vi "Mindsensors AngleSensor Config.vi"(10 "Node Data":T1, 11 "NXT":T2) -> ()   [LabVIEW 2010]
uses:
  <vilib>/NXT/Subs/LVHSConnector.ctl
  Datatypes/Node.ctl
  UI Controls/PlugInControls/Pluginbackground.ctl
  <vilib>/Utility/miscctls.llb/LVPointTypeDef.ctl
  <vilib>/NXT/Block Support/HWPage.SensorMode.ctl
  <vilib>/NXT/Block Support/HWPage.SensorType.ctl
  ConvertNodeAddrSensor.vi
panel:
  out "Raw Value (half degree)":i32
  out "RPM":i16
  in  "Device Addr":i32 format="%.0x"
  out "Angle (degrees)":i32
  out "?":u8
  out "number":i8
  in  "Device Address":string
  in  "NXT Port":string
  in  "Name":string
  out "Headline":string="Type (auto populated)"
  in  "Sensor Parameters":string
  in  "Instance Specific Data":cluster{"Example Data":dbl}
  in  "Reset":bool
  in  "Save":bool
  in  "Stop":bool
  out "Background":T3=TRUE
  # "Sensor Values"
  # "<- No controls below this line"
  # "Common controls such as Buttons, Rings, Sliders, Graphs, Decorations, etc can be found in the <labview>\\Targets\\NI\\NXT\\NXT Toolkit\\Schematic Editor\\UI Controls\\Plugin Controls\\ folder. Use these controls when possible to ensure a consistent look and feel with LabVIEW Education Edition."
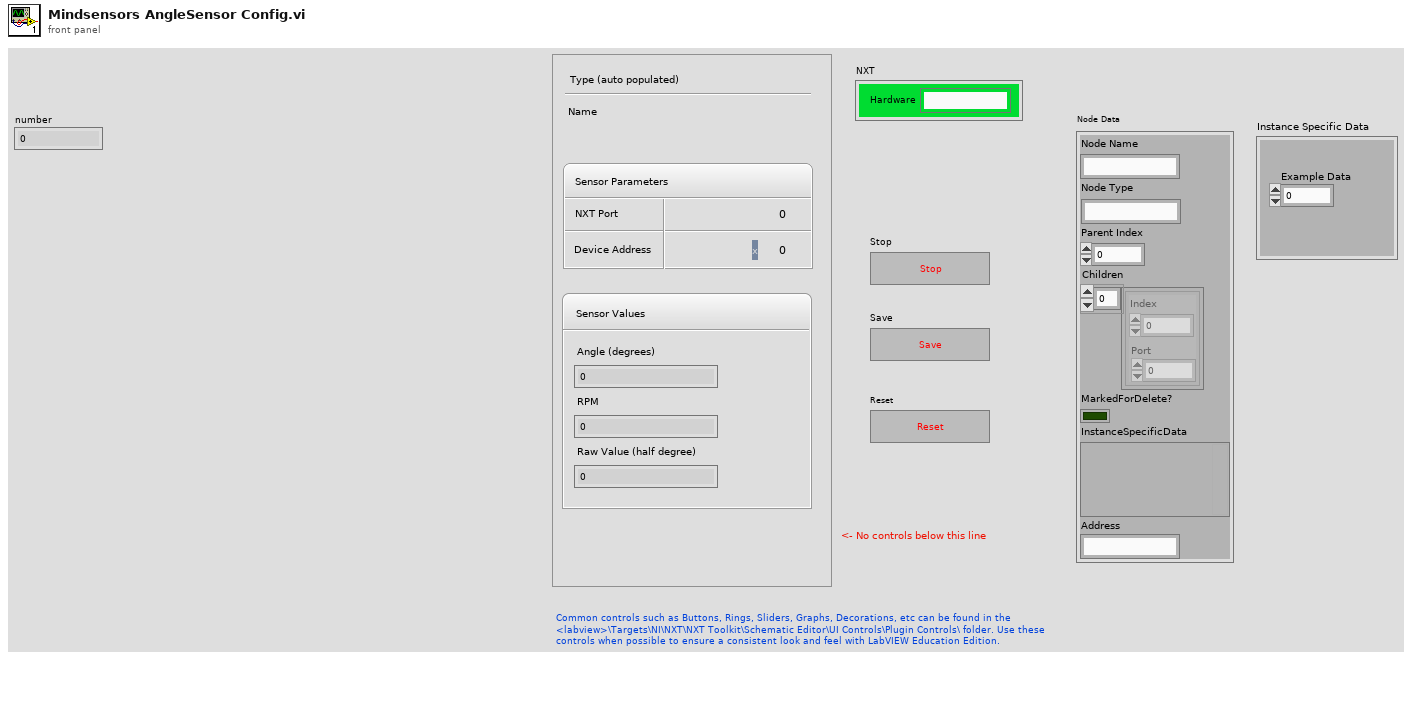
[diagram p1: front panel]
types:
  T1 = typedef "Node.ctl" = cluster{"Node Name":string, "Node Type":string, "Parent Index":i16, "Children":cluster{"Index":u16, "Port":u16}[], "MarkedForDelete?":bool, "InstanceSpecificData":variant, "Address":string}
  T2 = typedef "LVHSConnector.ctl" = cluster{"Hardware":string, "Flattened String":string}
  T3 = typedef "Pluginbackground.ctl" = bool
  T4 = typedef "LVPointTypeDef.ctl" = cluster{"Horizontal":i16, "Vertical":i16}
  T5 = enum8{"Enabled", "Disabled", "Disabled and Grayed Out"}
  T6 = typedef "HWPage.SensorMode.ctl" = u8
  T7 = typedef "HWPage.SensorType.ctl" = u8
  T8 = typedef "NXT_InputPort.ctl" = u8
  T9 = typedef "nxt.ctl" = cluster{"nxtHandle":u32, "fileHandle":u32, "fileIterHandle":u32, "moduleHandle":u32, "modIterHandle":u32, "nxtIterHandle":u32}
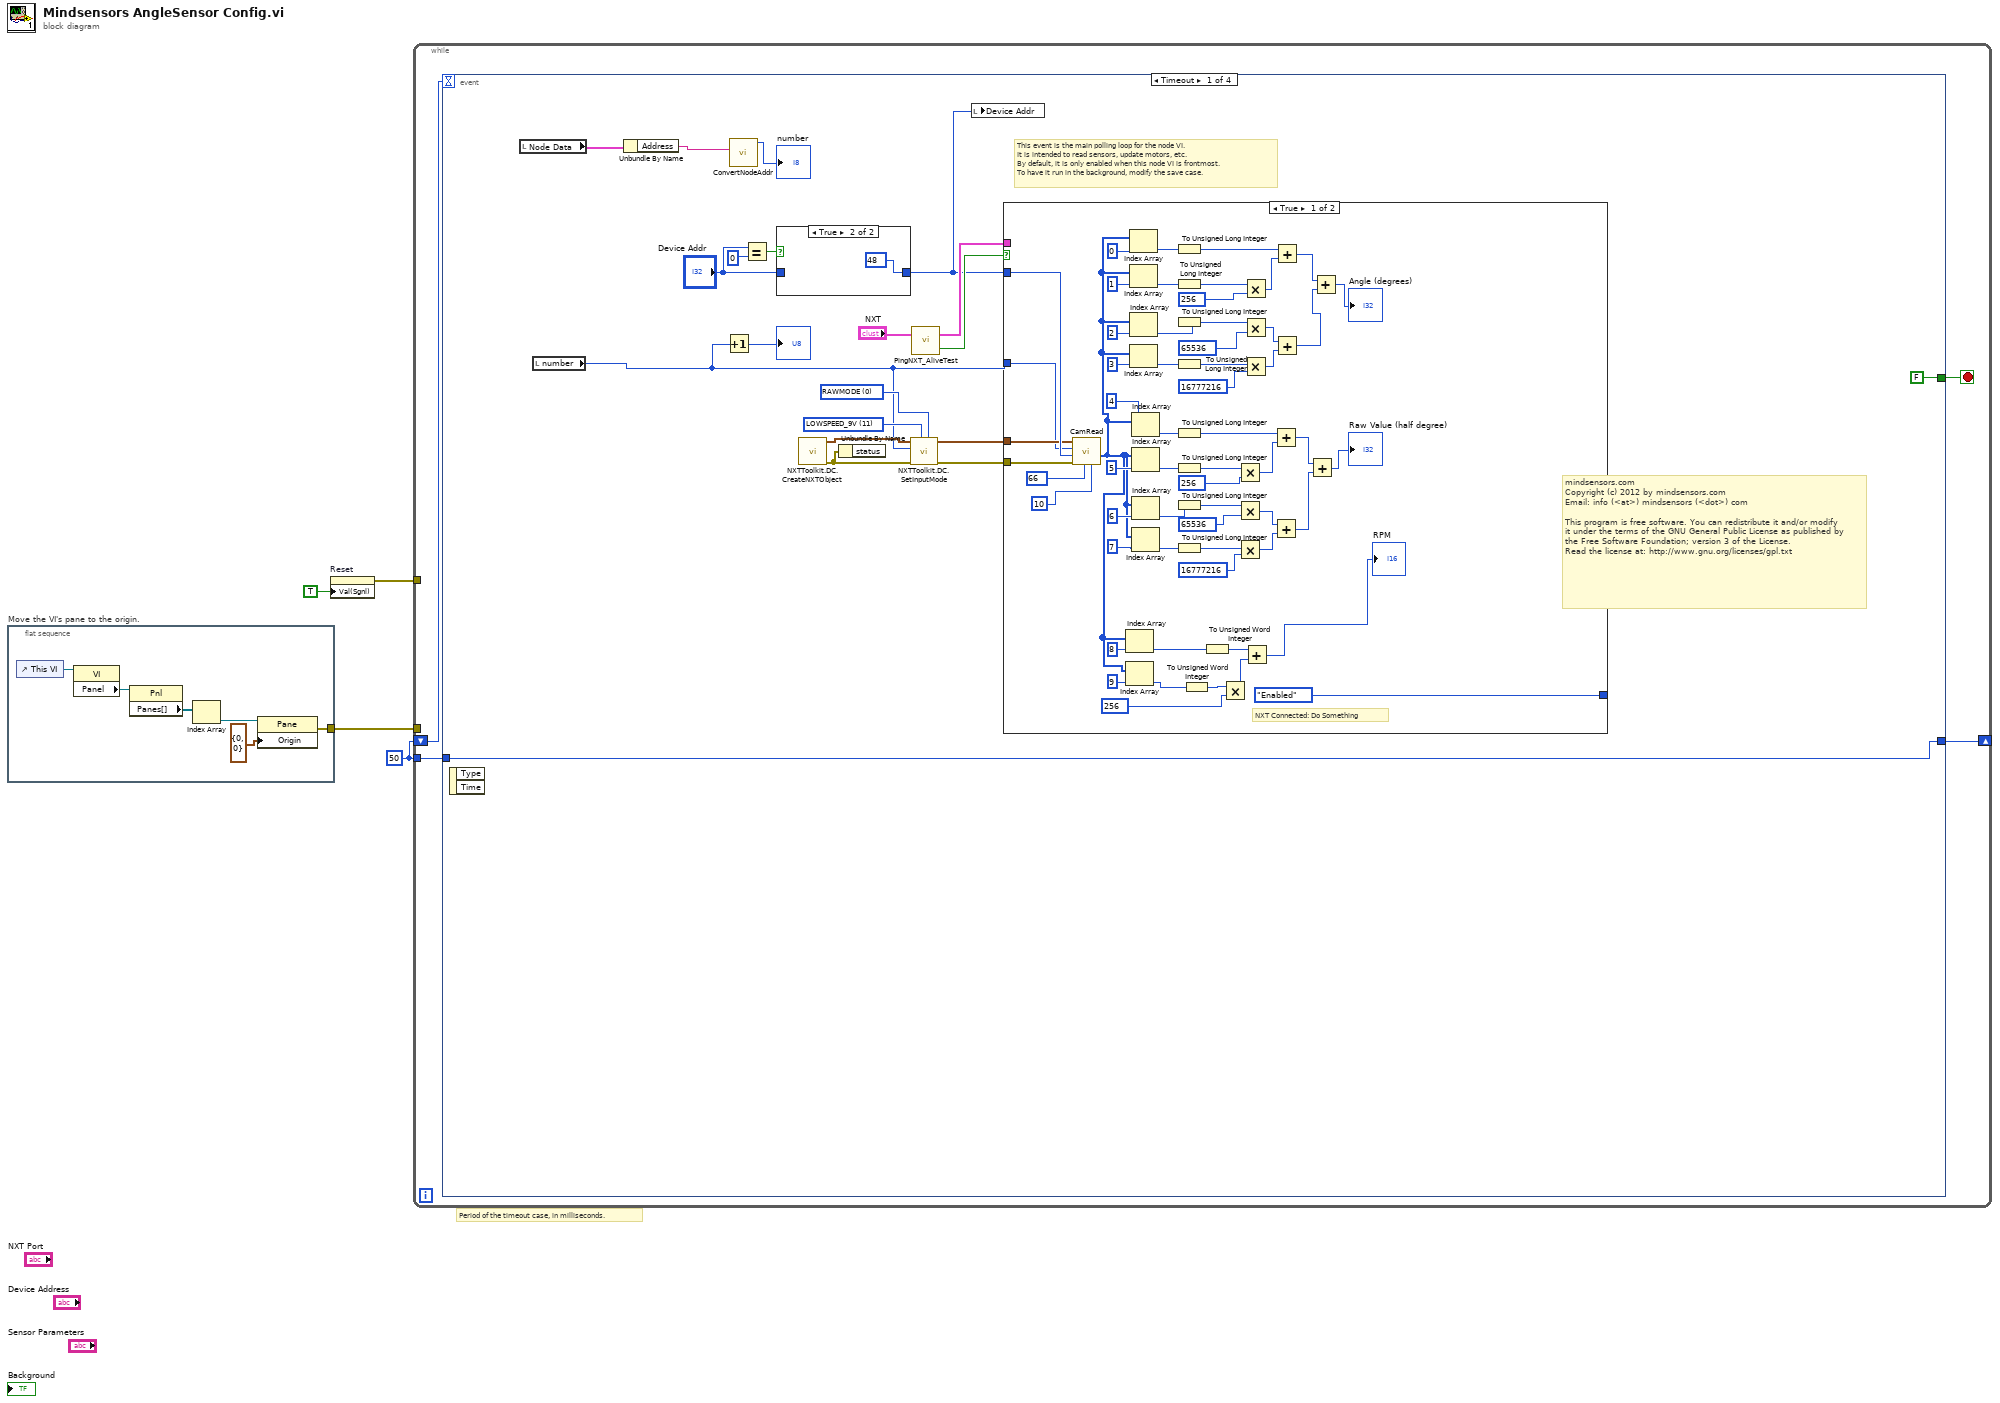
[diagram p0: block diagram]
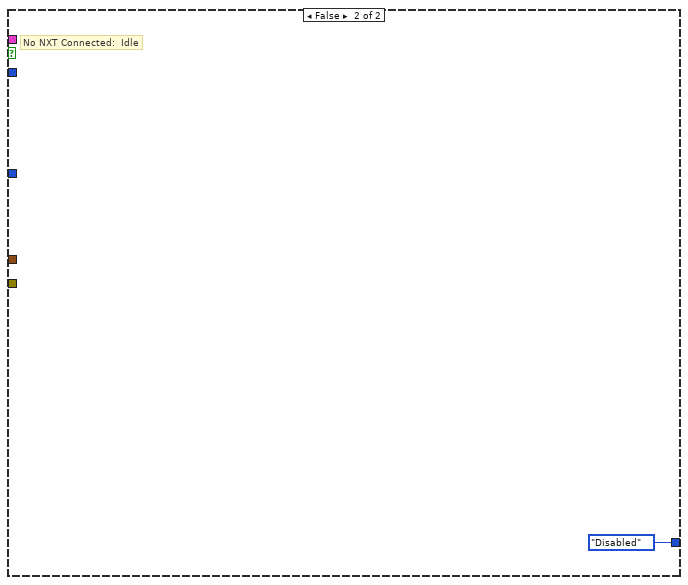
[diagram p3: hidden frame]
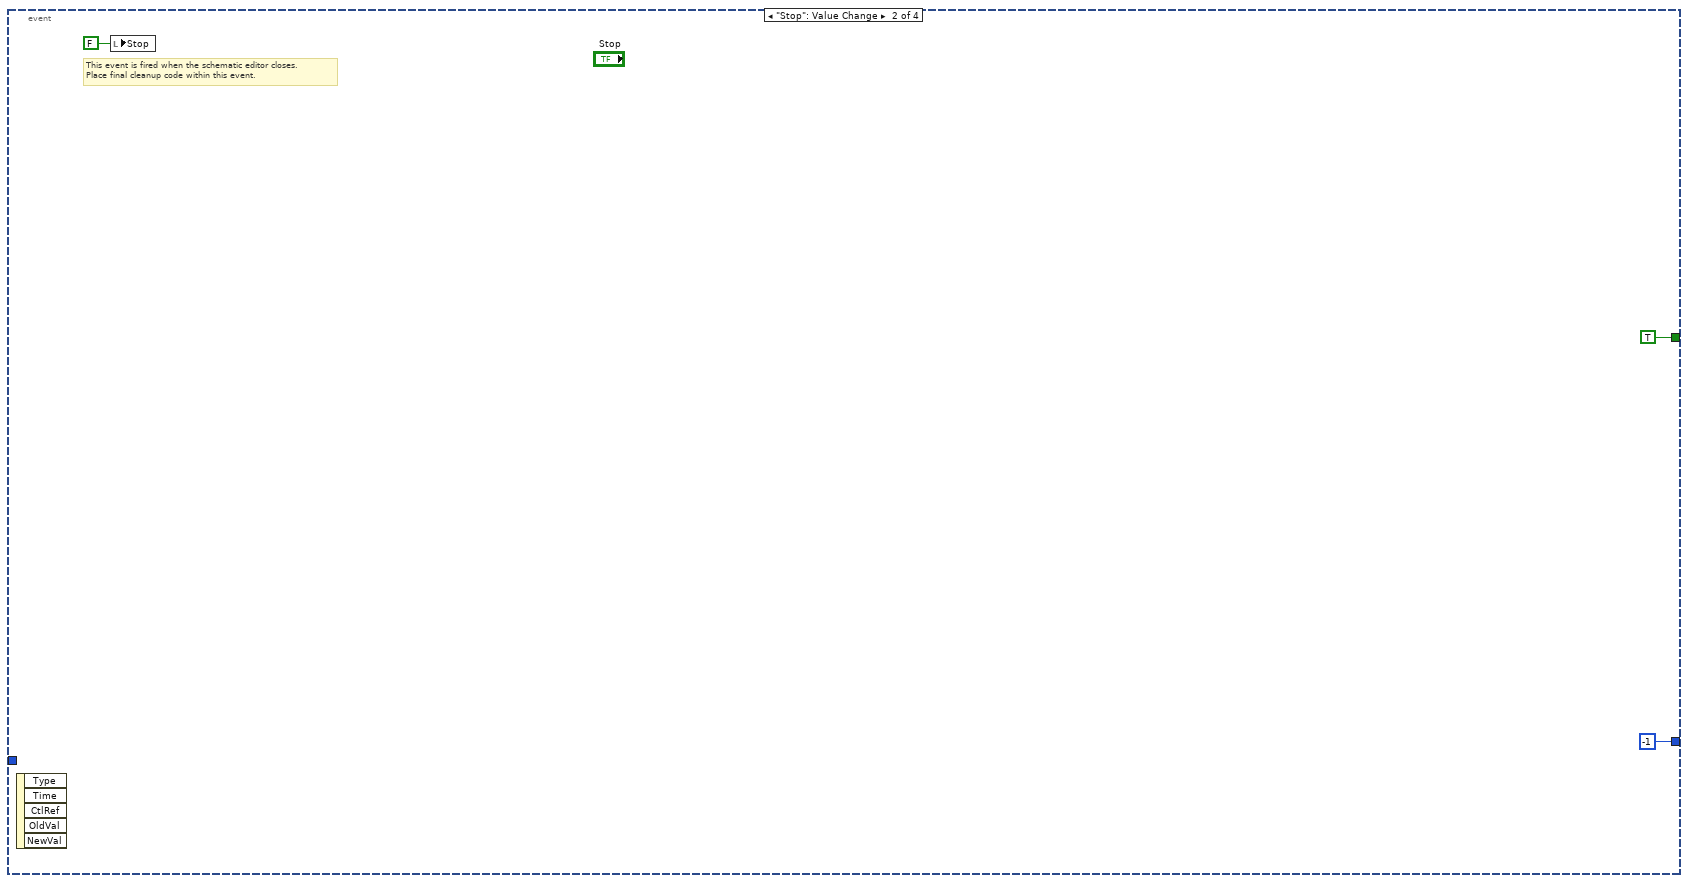
[diagram p4: hidden frame]
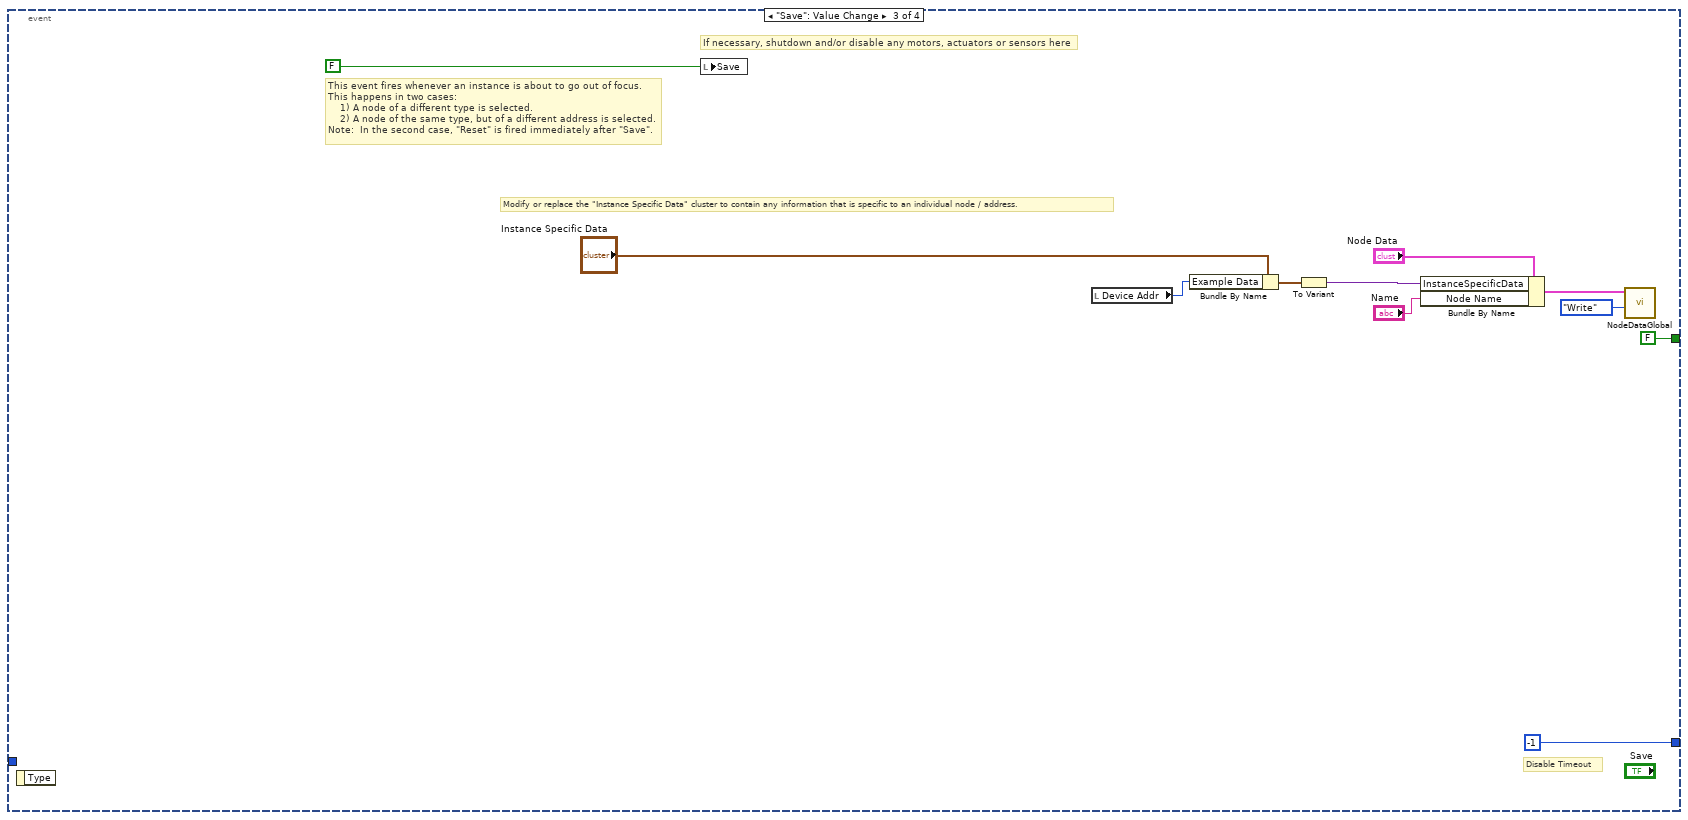
[diagram p5: hidden frame]
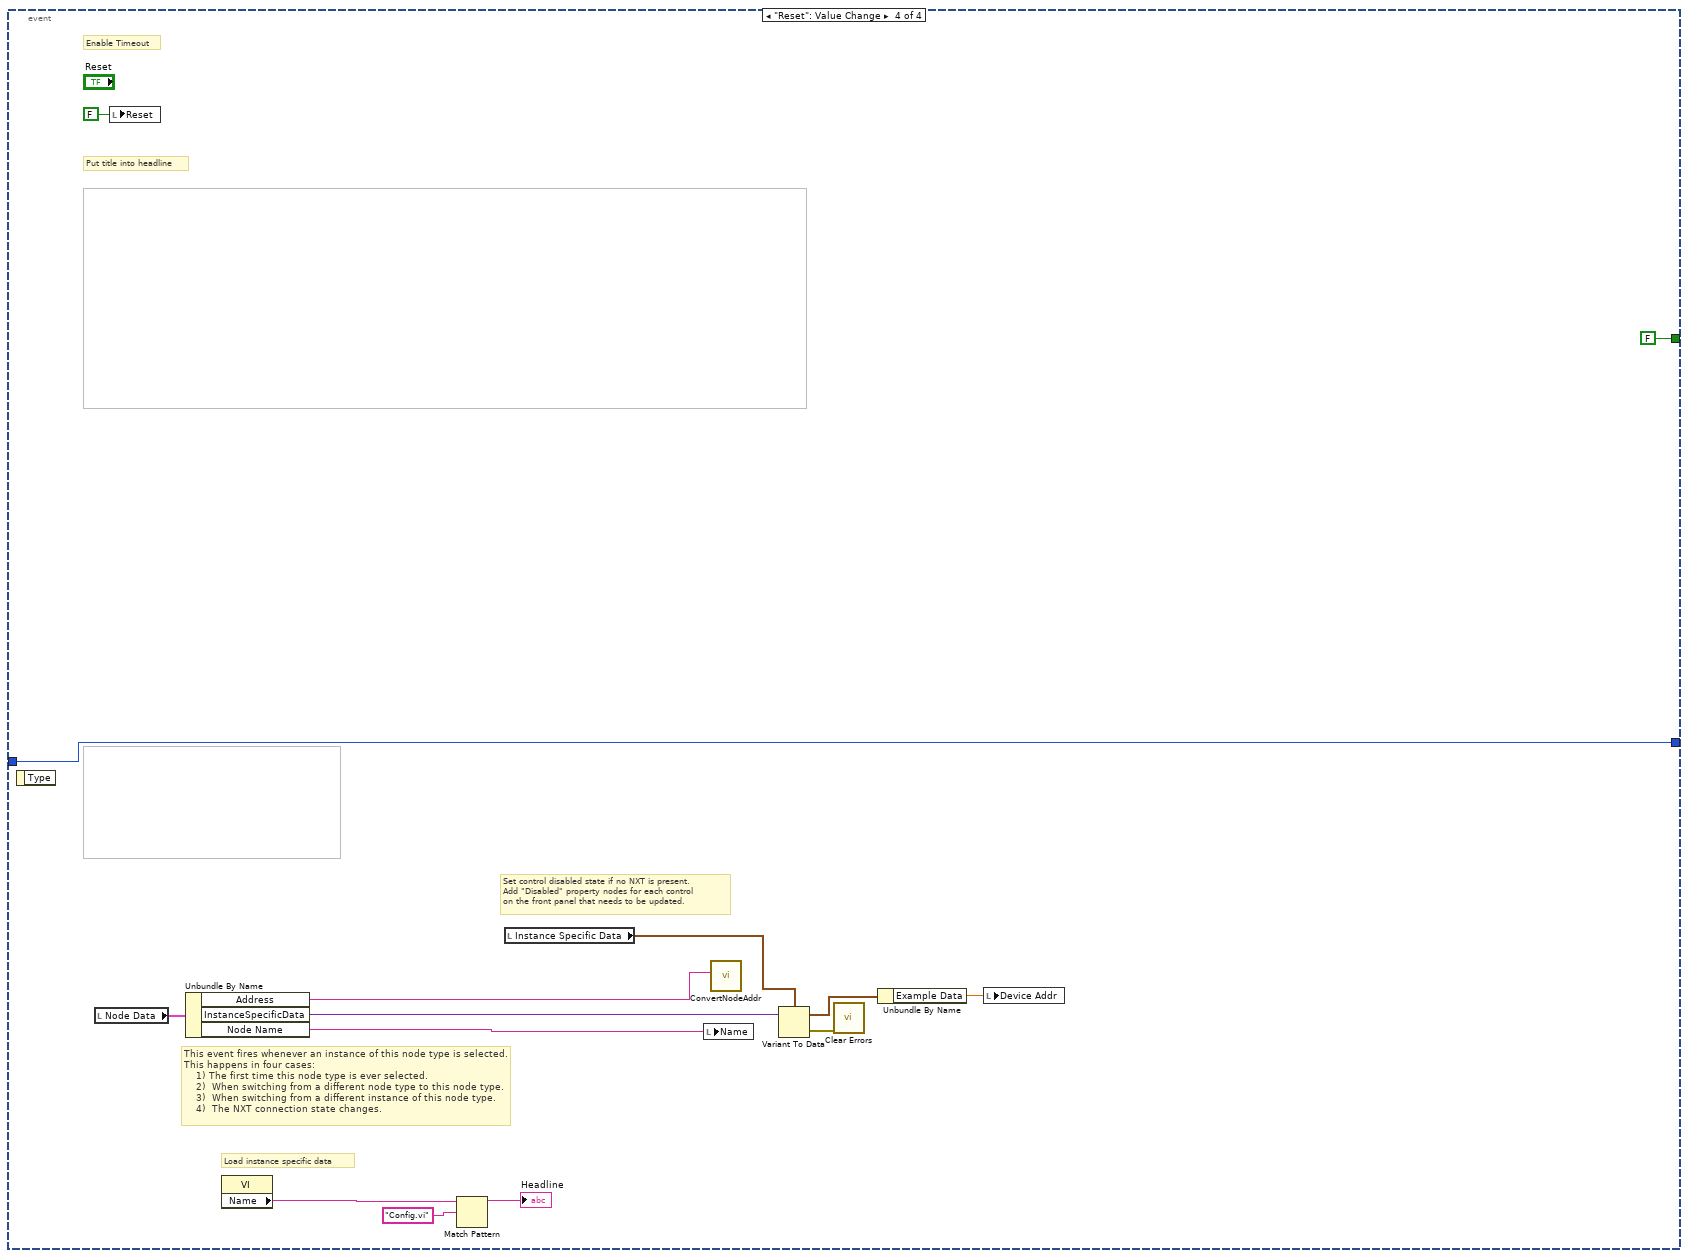
[diagram p6: hidden frame]
diagram:
  w2 = 50
  # "Period of the timeout case, in milliseconds."
  n1 = flat-sequence "Move the VI's pane to the origin." {
    tunnel: [w5] -> w1
    frame #0 {
      n2 = control-ref of="This VI"() -> (w6:refnum<vi>)
      n3 = property class="VI"(reference=w6) -> ("Panel"=w7:refnum<vi>)  [unwired: 1 in, 2 out]
      n4 = property class="Pnl"(reference=w7) -> ("Panes[]"=w8:refnum<vi>[])  [unwired: 1 in, 2 out]
      n5 = Index Array(array=w8) -> (element=w9:refnum<vi>)  [unwired: 1 in]
      n6 = property class="Pane"(reference=w9, "Origin"=T4 {"Horizontal"=0, "Vertical"=0}) -> (error out=w5:errorcluster)  [unwired: 1 in, 1 out]
    }
  }
  n7 = property on="Reset" class="Bool (strict)"("Val(Sgnl)"=TRUE ("Value (Signaling)")) -> (error out=w3:errorcluster)  [unwired: 2 in, 1 out]
  n8 = while {
    tunnel: w3 -> [_]
    shift-right: [w12] -> _
    shift-left: w2 -> [w13]
    tunnel: w2 -> [w11]
    tunnel: w1 -> [_]
    stop <- w14 stop-if-true
    n9 = event shown="[0] Timeout" {
      selector: _ -> [_ _ _ _]
      dyn-events: _ -> [_ _ _ _]
      timeout: w13 -> [_ _ _ _]
      tunnel: [FALSE TRUE FALSE FALSE] -> w14
      tunnel: [w33 -1 -1 w120] -> w12
      tunnel: w11 -> [w33 _ _ w120]
      event Timeout {
        w28 = T6 0 items=["RAWMODE"=0, "BOOLEANMODE"=32, "TRANSITIONCNTMODE"=64, "PERIODCOUNTERMODE"=96, "PCTFULLSCALEMODE"=128, "CELSIUSMODE"=160, "FAHRENHEITMODE"=192, "ANGLESTEPMODE"=224] ("Sensor Mode (RAWMODE)")
        w27 = T7 11 items=["NO_SENSOR", "SWITCH", "TEMPERATURE", "REFLECTION", "ANGLE", "LIGHT_ACTIVE", "LIGHT_INACTIVE", "SOUND_DB", "SOUND_DBA", "CUSTOM", "LOWSPEED", "LOWSPEED_9V", "HIGHSPEED"] ("Sensor Type (NO_SENSOR)")
        # "mindsensors.com\nCopyright (c) 2012 by mindsensors.com\nEmail: info (<at>) mindsensors (<dot>) com\n\nThis program is free software. You can redistribute it and/or modify\nit under the terms of the GNU General Public License as published by\nthe Free Software Foundation; version 3 of the License.\nRead the license at: http://www.gnu.org/licenses/gpl.txt"
        # "This event is the main polling loop for the node VI.\nIt is intended to read sensors, update motors, etc.\nBy default, it is only enabled when this node VI is frontmost.\nTo have it run in the background, modify the save case."
        n10 = event-data() -> ()  [unwired: 1 in, 2 out]
        n11 = local read "Node Data"() -> (w31:T1)
        n12 = local read "number"() -> (w16:i8)
        n13 = Unbundle By Name(w31) -> ("Address"=w18:string)
        n14 = Increment(x=w16) -> (x+1=→"?":i8)
        n15 = call-poly "ConvertNodeAddr.vi"("Sensor Port"=w18) -> ("NXT Port"=→"number":T8)  [unwired: 6 in, 4 out]
        n16 = Equal?(x="Device Addr", y=u8 0) -> (x = y?=w21:bool)
        n17 = case shown="True" w21 {
          tunnel: [w35 u8 48 ("Device Addr 2")] -> w20
          tunnel: "Device Addr" -> [w35 _]
          frame False {
          }
          frame True {
          }
        }
        n18 = call <vilib>:"NXTToolkit.DC.CreateNXTObject.vi"() -> ("error out"=w25:errorcluster, "NXTObject"=w26:T9)  [unwired: 9 in, 1 out]
        n19 = Unbundle By Name(w25) -> ()  [unwired: 1 out]
        n20 = call <vilib>:"NXTToolkit.DC.SetInputMode.vi"("Sensor Mode (RAWMODE)"=w28, "Sensor Type (NO_SENSOR)"=w27, "error in (no error)"=w25, "Input Port (Port 1)"=w16, "NXTObject"=w26) -> ("error out"=w23:errorcluster, "NXTObject dup"=w24:T9)  [unwired: 4 in, 1 out]
        n21 = call <vilib>:"PingNXT_AliveTest.vi"("NXT"="NXT") -> ("connected?"=w30:bool, "NXT"=w29:T2)  [unwired: 1 in]
        n22 = local write "Device Addr"(w20) -> ()
        n23 = case shown="True" w30 {
          tunnel: [T5."Enabled" ("Disabled") T5."Disabled" ("Disabled")] -> _
          tunnel: w29 -> [_ _]
          tunnel: w24 -> [w91 _]
          tunnel: w23 -> [w90 _]
          tunnel: w16 -> [w89 _]
          tunnel: w20 -> [w93 _]
          frame True {
            # "NXT Connected: Do Something"
            n24 = call <vilib>:"CamRead.vi"("bytes to read"=u8 10, "Reg Address"=u8 66, "error in (no error)"=w90, "Device Address"=w93, "Input Port in"=w89, "NXTObject"=w91) -> ("data Buffer"=w43:u8[])  [unwired: 5 out]
            n25 = Index Array(array=w43, index=8) -> (element=w86:u8)
            n26 = Index Array(array=w43, index=9) -> (element=w84:u8)
            n27 = Index Array(array=w43, index=0) -> (element=w66:u8)
            n28 = Index Array(array=w43, index=1) -> (element=w75:u8)
            n29 = Index Array(array=w43, index=2) -> (element=w74:u8)
            n30 = Index Array(array=w43, index=3) -> (element=w73:u8)
            n31 = Index Array(array=w43, index=4) -> (element=w46:u8)
            n32 = Index Array(array=w43, index=5) -> (element=w57:u8)
            n33 = Index Array(array=w43, index=6) -> (element=w55:u8)
            n34 = Index Array(array=w43, index=7) -> (element=w54:u8)
            n35 = To Unsigned Long Integer(number=w66) -> (unsigned 32bit integer=w72:u32)
            n36 = To Unsigned Long Integer(number=w75) -> (unsigned 32bit integer=w71:u32)
            n37 = To Unsigned Long Integer(number=w74) -> (unsigned 32bit integer=w69:u32)
            n38 = To Unsigned Long Integer(number=w73) -> (unsigned 32bit integer=w70:u32)
            n39 = To Unsigned Long Integer(number=w46) -> (unsigned 32bit integer=w53:u32)
            n40 = To Unsigned Long Integer(number=w57) -> (unsigned 32bit integer=w52:u32)
            n41 = To Unsigned Long Integer(number=w55) -> (unsigned 32bit integer=w50:u32)
            n42 = To Unsigned Long Integer(number=w54) -> (unsigned 32bit integer=w51:u32)
            n43 = To Unsigned Word Integer(number=w84) -> (unsigned 16bit integer=w44:u16)
            n44 = To Unsigned Word Integer(number=w86) -> (unsigned 16bit integer=w45:u16)
            n45 = Multiply(x=w44, y=256) -> (x*y=w85:i32)
            n46 = Multiply(x=w52, y=u32 256) -> (x*y=w63:u32)
            n47 = Multiply(x=w50, y=u32 65536) -> (x*y=w49:u32)
            n48 = Multiply(x=w51, y=u32 16777216) -> (x*y=w61:u32)
            n49 = Multiply(x=w71, y=u32 256) -> (x*y=w81:u32)
            n50 = Multiply(x=w69, y=u32 65536) -> (x*y=w68:u32)
            n51 = Multiply(x=w70, y=u32 16777216) -> (x*y=w79:u32)
            n52 = Add(x=w45, y=w85) -> (x+y=→"RPM":i32)
            n53 = Add(x=w53, y=w63) -> (x+y=w56:u32)
            n54 = Add(x=w49, y=w61) -> (x+y=w47:u32)
            n55 = Add(x=w72, y=w81) -> (x+y=w38:u32)
            n56 = Add(x=w68, y=w79) -> (x+y=w39:u32)
            n57 = Add(x=w56, y=w47) -> (x+y=→"Raw Value (half degree)":u32)
            n58 = Add(x=w38, y=w39) -> (x+y=→"Angle (degrees)":u32)
          }
          frame False {
            # "No NXT Connected:  Idle"
          }
        }
      }
      event "Stop": Value Change {
        # "This event is fired when the schematic editor closes.\nPlace final cleanup code within this event."
        n59 = event-data() -> ()  [unwired: 1 in, 5 out]
        n60 = local write "Stop"(FALSE ("stop")) -> ()
      }
      event "Save": Value Change {
        # "If necessary, shutdown and/or disable any motors, actuators or sensors here"
        # "Modify or replace the \"Instance Specific Data\" cluster to contain any information that is specific to an individual node / address."
        # "Disable Timeout"
        # "This event fires whenever an instance is about to go out of focus.\nThis happens in two cases:\n    1) A node of a different type is selected.\n    2) A node of the same type, but of a different address is selected.\nNote:  In the second case, \"Reset\" is fired immediately after \"Save\"."
        n61 = event-data() -> ()  [unwired: 1 in, 1 out]
        n62 = local write "Save"(FALSE ("stop")) -> ()
        n63 = local read "Device Addr"() -> (w100:i32)
        n64 = Bundle By Name(cluster="Instance Specific Data", "Example Data"=w100) -> (w101:cluster{"Example Data":dbl})
        n65 = To Variant(anything=w101) -> (Variant=w108:variant)
        n66 = Bundle By Name(cluster="Node Data", "InstanceSpecificData"=w108, "Node Name"="Name") -> (w107:T1)
        n67 = call "NodeDataGlobal.vi"("Action"=enum16{"Read", "Write"}."Write", "Node Data In"=w107) -> ()  [unwired: 8 in, 2 out]
      }
      event "Reset": Value Change {
        # "Set control disabled state if no NXT is present.\nAdd \"Disabled\" property nodes for each control\non the front panel that needs to be updated."
        # "Load instance specific data"
        # "Enable Timeout"
        # "This event fires whenever an instance of this node type is selected.\nThis happens in four cases:\n    1) The first time this node type is ever selected.\n    2)  When switching from a different node type to this node type.\n    3)  When switching from a different instance of this node type. \n    4)  The NXT connection state changes."
        # "Put title into headline"
        n68 = event-data() -> ()  [unwired: 1 in, 1 out]
        n69 = local read "Node Data"() -> (w121:T1)
        n70 = local write "Reset"(FALSE ("Reset")) -> ()
        n71 = Unbundle By Name(w121) -> ("Address"=w112:string, "InstanceSpecificData"=w122:variant, "Node Name"=w114:string)
        n72 = property class="VI"() -> ("Name"=w116:string)  [unwired: 2 in, 2 out]
        n73 = Match Pattern(string=w116, regular expression="Config.vi") -> (before substring=→"Headline":string)  [unwired: 1 in, 3 out]
        n74 = local read "Instance Specific Data"() -> (w119:cluster{"Example Data":dbl})
        n75 = local write "Name"(w114) -> ()
        n76 = call-poly "ConvertNodeAddr.vi"("Sensor Port"=w112) -> ()  [unwired: 6 in, 5 out]
        n77 = Variant To Data(Variant=w122, type=w119) -> (error out=w118:errorcluster, data=w113:cluster{"Example Data":dbl})  [unwired: 1 in]
        n78 = call <vilib>:"Clear Errors.vi"("error in (no error)"=w118) -> ()  [unwired: 6 in, 1 out]
        n79 = Unbundle By Name(w113) -> ("Example Data"=w111:dbl)
        n80 = local write "Device Addr"(w111) -> ()
      }
    }
  }
